vi "FlatToRichniswitch_grpc_CanConnectResponse.vi"(5 "OutputClusterType":T1, 11 "InputCluster":T3) -> (3 "OutputCluster":T1)   [LabVIEW 2021, in "NI Switch_client.lvlib"]
uses:
  NI Switch_client.lvlib
  niswitch_grpc_CanConnectResponse_Flat.ctl
  niswitch_grpc_PathCapability.ctl
  niswitch_grpc_CanConnectResponse.ctl
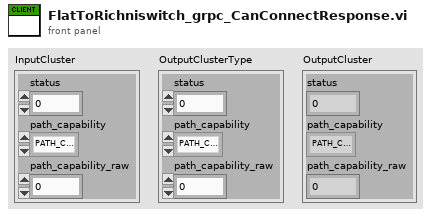
[diagram p1: front panel]
types:
  T1 = typedef "NI Switch_client.lvlib/niswitch_grpc_CanConnectResponse.ctl" = cluster{"status":i32, "path_capability":T2, "path_capability_raw":i32}
  T2 = typedef "NI Switch_client.lvlib/niswitch_grpc_PathCapability.ctl" = enum32{"PATH_CAPABILITY_UNSPECIFIED", "PATH_CAPABILITY_NISWITCH_VAL_PATH_AVAILABLE", "PATH_CAPABILITY_NISWITCH_VAL_PATH_EXISTS", "PATH_CAPABILITY_NISWITCH_VAL_PATH_UNSUPPORTED", "PATH_CAPABILITY_NISWITCH_VAL_RESOURCE_IN_USE", "PATH_CAPABILITY_NISWITCH_VAL_SOURCE_CONFLICT", "PATH_CAPABILITY_NISWITCH_VAL_CHANNEL_NOT_AVAILABLE"}
  T3 = typedef "NI Switch_client.lvlib/niswitch_grpc_CanConnectResponse_Flat.ctl" = cluster{"status":i32, "path_capability":T2, "path_capability_raw":i32}
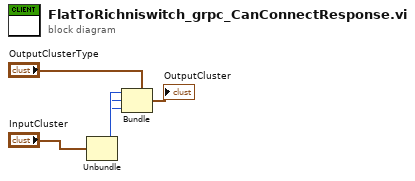
[diagram p0: block diagram]
diagram:
  n1 = Unbundle "Unbundle"("InputCluster") -> ("status"=w3:i32, "path_capability"=w2:T2, "path_capability_raw"=w1:i32)
  n2 = Bundle "Bundle"(cluster="OutputClusterType", "status"=w3, "path_capability"=w2, "path_capability_raw"=w1) -> (→"OutputCluster":T1)
